vi "调试记录插入.vi"(9 "内容":string, 11 "调试记录":refnum<vi>) -> ()   [LabVIEW 2013]
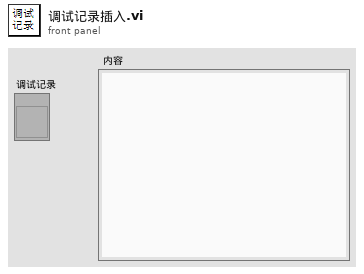
[diagram p1: front panel]
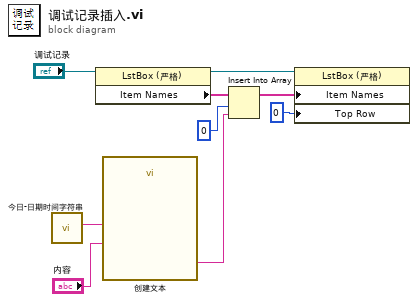
[diagram p0: block diagram]
diagram:
  n1 = call "今日-日期时间字符串.vi"() -> ("hh:mm:ss"=w9:string)  [unwired: 9 in, 2 out]
  n2 = property on="属性节点" class="LstBox (严格)"(reference="调试记录") -> (reference out=w3:refnum<vi>, "Item Names"=w5:string[])  [unwired: 1 in, 1 out]
  n3 = call "创建文本"("时间"=w9, "内容"="内容") -> ("Result"=w1:string)  [unwired: 12 in, 1 out]
  n4 = Insert Into Array(array=w5, index=0 ("索引"), new element=w1) -> (w7:string[])
  n5 = property on="属性节点" class="LstBox (严格)"(reference=w3, "Item Names"=w7, "Top Row"=0 ("顶行")) -> ()  [unwired: 1 in, 2 out]
